vi "14.1 State Programming.vi"() -> ()   [LabVIEW 2019]
uses:
  13.1 DAQmx Configuration Cluster.ctl
  13.1 Weather Data.ctl
  14.1 Begining State.ctl
  <vilib>/DAQmx/read.llb/DAQmx Read (Analog DBL 1Chan 1Samp).vi
  <vilib>/DAQmx/create/channels.llb/DAQmx Create Channel (AI-Temperature-Thermocouple).vi
  <vilib>/DAQmx/miscellaneous.llb/DAQmx Fill In Error Info.vi
panel:
  in  "Stop":bool
  out "Warning":string
  in  "Lower limit":dbl
  in  "Upper limit":dbl
  out "Temperature History":dbl format="%0.2f"
  in  "DAQmx Configuration Cluster":T1={"Desired Sample Rate (Hz)"=-1.0, "sample mode"=10178, "Minimum value"=-1.0, "Maximum value"=-1.0, "Thermocouple Channel"="", "units"=10143, "thermocouple type"=10072} {"thermocouple type" items=["J"=10072, "K"=10073, "N"=10077, "R"=10082, "S"=10085, "T"=10086, "B"=10047, "E"=10055]; "units" items=["Deg C"=10143, "Deg F"=10144, "Kelvins"=10325, "Deg R"=10145, "From Custom Scale"=10065]; "sample mode" items=["Finite Samples"=10178, "Continuous Samples"=10123, "Hardware Timed Single Point"=12522]}
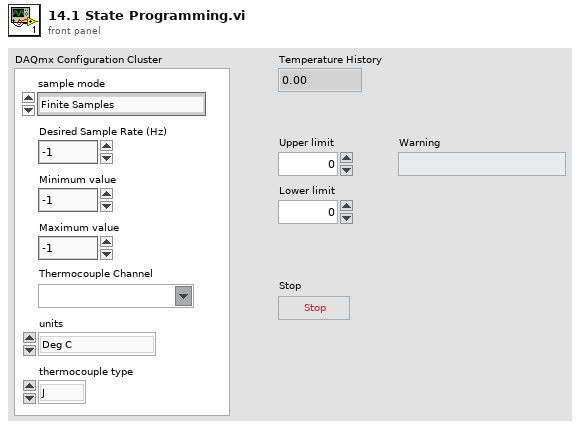
[diagram p1: front panel]
types:
  T1 = typedef "13.1 DAQmx Configuration Cluster.ctl" = cluster{"Desired Sample Rate (Hz)":dbl, "sample mode":i32, "Minimum value":dbl, "Maximum value":dbl, "Thermocouple Channel":tag, "units":i32, "thermocouple type":i32}
  T2 = typedef "14.1 Begining State.ctl" = enum16{"Initialize", "Acquire", "Analyze", "Log", "Check time", "Shutdown"}
  T3 = enum16{"open", "replace", "create", "open or create", "replace or create", "replace or create with confirmation"}
  T4 = typedef "13.1 Weather Data.ctl" = cluster{"Current Temperature":dbl, "Max Temperature":dbl, "Min Temperature":dbl, "Warning?":bool, "Warning text":string}
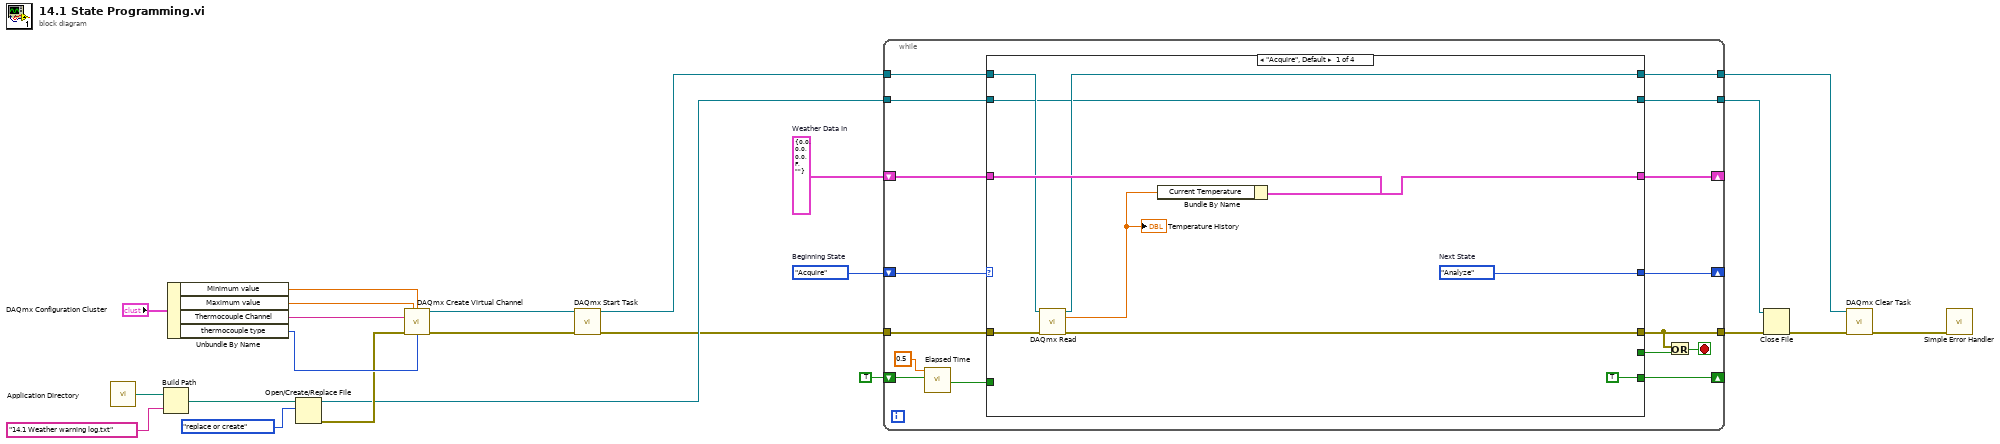
[diagram p0: block diagram]
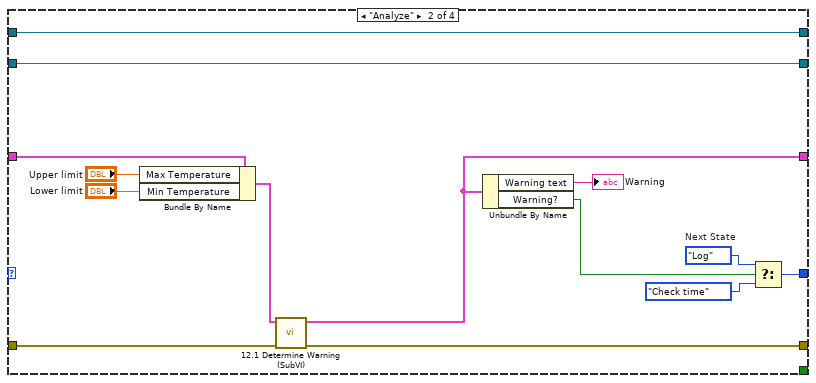
[diagram p2: hidden frame]
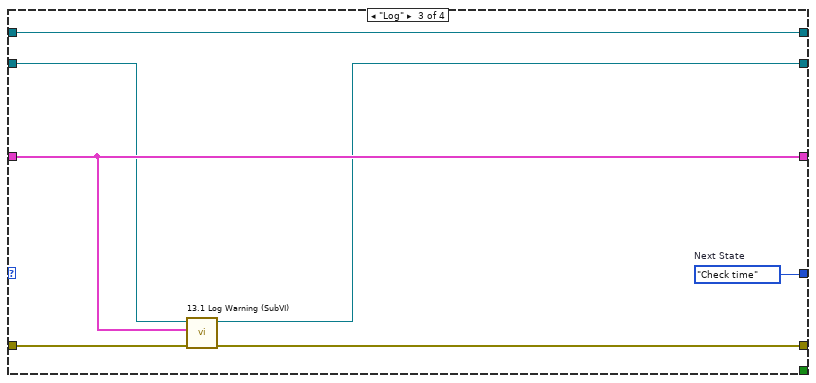
[diagram p3: hidden frame]
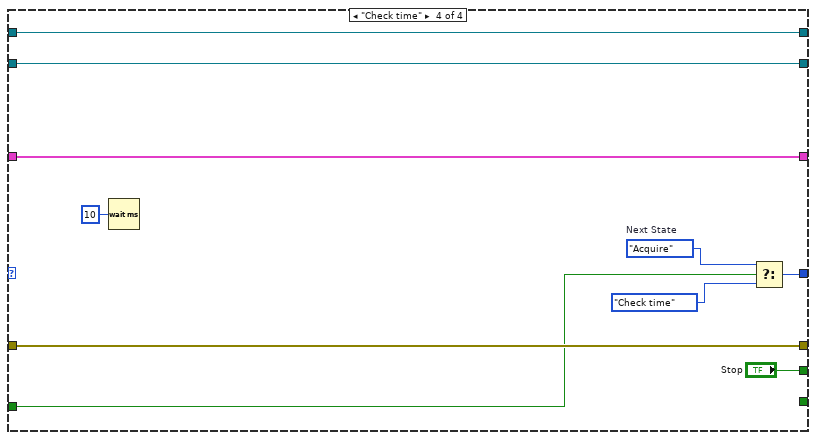
[diagram p4: hidden frame]
diagram:
  w7 = 14.1_Begining_State."Acquire"  # Beginning State
  w8 = T4 {"Current Temperature"=0.0, "Max Temperature"=0.0, "Min Temperature"=0.0, "Warning?"=FALSE, "Warning text"=""}  # Weather Data In
  n1 = call <vilib>:"Application Directory.vi"() -> ("Application Directory"=w20:path)
  n2 = Build Path(base path=w20, name or relative path="14.1 Weather warning log.txt") -> (appended path=w22:path)
  n3 = Unbundle By Name("DAQmx Configuration Cluster") -> ("Minimum value"=w16:dbl, "Maximum value"=w14:dbl, "Thermocouple Channel"=w15:tag, "thermocouple type"=w13:i32)
  n4 = Open/Create/Replace File(file path (use dialog)=w22, operation (0:open)=T3."replace or create") -> (refnum out=w10:refnum<file>, error out=w12:errorcluster)  [unwired: 4 in, 1 out]
  n5 = call-poly <vilib>:"DAQmx Create Virtual Channel.vi"("maximum value"=w14, "minimum value"=w16, "physical channels"=w15, "error in"=w12, "thermocouple type"=w13) -> ("task out"=w18:refnum<k21>, "error out"=w17:errorcluster)  [unwired: 9 in]
  n6 = call <vilib>:"DAQmx Start Task.vi"("task/channels in"=w18, "error in"=w17) -> ("task out"=w11:refnum<k21>, "error out"=w9:errorcluster)  [unwired: 12 in]
  n7 = while {
    tunnel: w11 -> [w33]
    tunnel: w10 -> [w34]
    tunnel: w9 -> [w35]
    shift-right: [w36] -> _
    shift-left: w8 -> [w37]
    shift-right: [w38] -> _
    shift-left: w7 -> [w39]
    tunnel: [w32] -> w2
    shift-right: [w27] -> _
    shift-left: TRUE -> [w30]
    tunnel: [w26] -> w4
    tunnel: [w25] -> w5
    stop <- w28 stop-if-true
    n8 = call "Elapsed Time"("Time Target (s)"=0.5, "Reset"=w30) -> ("Time has Elapsed"=w29:bool)  [unwired: 10 in, 7 out]
    n9 = case shown="\"Acquire\", Default" w39 {
      tunnel: [w49 w55 w65 w76] -> w38
      tunnel: w37 -> [w48 w63 w69 w79]
      tunnel: [w47 w57 w69 w79] -> w36
      tunnel: w35 -> [w46 w60 w70 w72]
      tunnel: w34 -> [w40 w50 w68 w78]
      tunnel: w33 -> [w45 w51 w66 w77]
      tunnel: [w44 w51 w66 w77] -> w32
      tunnel: w29 -> [_ _ _ w71]
      tunnel: [w42 w58 w64 w72] -> w25
      tunnel: [TRUE _ _ _] -> w27
      tunnel: [w40 w50 w67 w78] -> w26
      tunnel: [_ _ _ "Stop"] -> w24
      frame "Acquire", Default {
        w49 = 14.1_Begining_State."Analyze"  # Next State
        n10 = call-poly <vilib>:"DAQmx Read.vi"("task/channels in"=w45, "error in"=w46) -> ("task out"=w44:refnum<k21>, "data"=w43:dbl, "error out"=w42:errorcluster)  [unwired: 11 in]
        "Temperature History" <- w43
        n11 = Bundle By Name(cluster=w48, "Current Temperature"=w43) -> (w47:T4)
      }
      frame "Analyze" {
        w54 = 14.1_Begining_State."Log"  # Next State
        n12 = Bundle By Name(cluster=w63, "Max Temperature"="Upper limit", "Min Temperature"="Lower limit") -> (w59:T4)
        n13 = call "12.1 Determine Warning (SubVI).vi"("Error In"=w60, "Weather Data In"=w59) -> ("Error Out"=w58:errorcluster, "Weather Data Out"=w57:T4)  [unwired: 8 in]
        n14 = Unbundle By Name(w57) -> ("Warning text"=→"Warning":string, "Warning?"=w52:bool)
        n15 = Select(t=w54, s=w52, f=14.1_Begining_State."Check time" ("State")) -> (s? t:f=w55:T2)
      }
      frame "Log" {
        w65 = 14.1_Begining_State."Check time"  # Next State
        n16 = call "13.1 Log Warning (SubVI).vi"("Error In"=w70, "Weather Data In"=w69, "refnum in"=w68) -> ("Error Out"=w64:errorcluster, "refnum out"=w67:refnum<file>)  [unwired: 7 in]
      }
      frame "Check time" {
        w75 = 14.1_Begining_State."Acquire"  # Next State
        n17 = Wait (ms)(milliseconds to wait=u32 10) -> ()  [unwired: 1 out]
        n18 = Select(t=w75, s=w71, f=14.1_Begining_State."Check time" ("Next State")) -> (s? t:f=w76:T2)
      }
    }
    n19 = Or(x=w25, y=w24) -> (x .or. y?=w28:bool)
  }
  n20 = Close File(refnum=w4, error in=w5) -> (error out=w3:errorcluster)  [unwired: 1 out]
  n21 = call <vilib>:"DAQmx Clear Task.vi"("task in"=w2, "error in"=w3) -> ("error out"=w1:errorcluster)  [unwired: 13 in]
  n22 = call <vilib>:"Simple Error Handler.vi"("error in (no error)"=w1) -> ()  [unwired: 4 in, 5 out]
